vi "BreadBoardLabVIEWtoArduino.vi"() -> ()   [LabVIEW 2024]
uses:
  <vilib>/Instr/_visa.llb/VISA Configure Serial Port (Instr).vi
  <vilib>/Utility/file.llb/Write Delimited Spreadsheet (DBL).vi
  <vilib>/Utility/file.llb/Write Delimited Spreadsheet (string).vi
panel:
  in  "Numeric 2":dbl
  out "Numeric":dbl format="%#_6f"
  in  "file path (dialog if empty)":path
  out "x-y":u32
  out "String":string
  in  "Boolean":bool
  in  "stop":bool
  in  "VISA resource name":refnum<visa-resource-name>
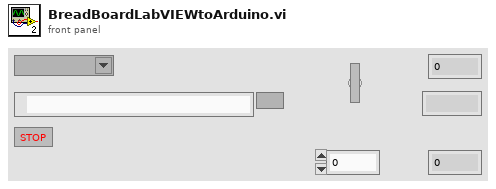
[diagram p1: front panel]
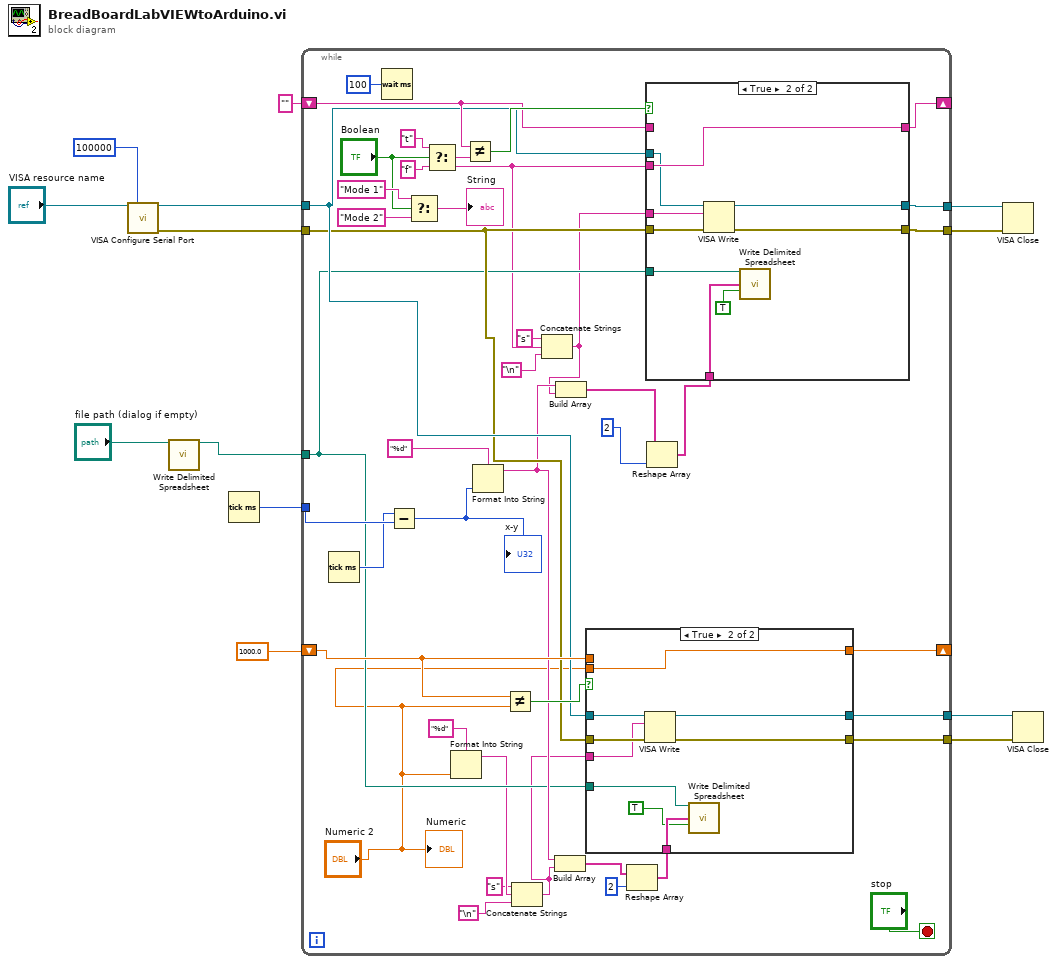
[diagram p0: block diagram]
diagram:
  n1 = call-poly "VISA Configure Serial Port"("VISA resource name"="VISA resource name", "timeout (10sec)"=u32 100000) -> ("VISA resource name out"=w2:refnum<visa-resource-name>, "error out"=w1:errorcluster)  [unwired: 12 in]
  n2 = call-poly <vilib>:"Write Delimited Spreadsheet.vi"("file path (dialog if empty)"="file path (dialog if empty)") -> ("new file path (Not A Path if cancelled)"=w8:path)  [unwired: 13 in, 1 out]
  n3 = Tick Count (ms)() -> (millisecond timer value=w7:u32)
  n4 = while {
    tunnel: w1 -> [w28]
    tunnel: [w48] -> w11
    tunnel: [w47] -> w10
    tunnel: w2 -> [w31]
    shift-right: [w49] -> _
    shift-left: "" -> [w50]
    tunnel: w8 -> [w23]
    tunnel: w7 -> [w40]
    shift-right: [w35] -> _
    shift-left: 1000.0 -> [w34]
    tunnel: [w30] -> w4
    tunnel: [w29] -> w3
    stop <- "stop" stop-if-true
    n5 = Tick Count (ms)() -> (millisecond timer value=w39:u32)
    n6 = Wait (ms)(milliseconds to wait=u32 100) -> ()  [unwired: 1 out]
    n7 = Subtract(x=w39, y=w40) -> (x-y=w41:u32)
    "x-y" <- w41
    n8 = Select(t="Mode 1", s="Boolean", f="Mode 2") -> (s? t:f=→"String":string)
    n9 = Select(t="t", s="Boolean", f="f") -> (s? t:f=w20:string)
    n10 = Format Into String(format string="%d", "Numeric 2") -> (resulting string=w18:string)  [unwired: 2 in, 1 out]
    n11 = Not Equal?(x=w50, y=w20) -> (x != y?=w53:bool)
    n12 = Format Into String(format string="%d", w41) -> (resulting string=w26:string)  [unwired: 2 in, 1 out]
    n13 = Not Equal?(x=w34, y="Numeric 2") -> (x != y?=w33:bool)
    n14 = Concatenate Strings("s" ("string"), w18, "\n") -> (w17:string)
    n15 = Concatenate Strings("s" ("string"), w20, "\n") -> (w21:string)
    n16 = Build Array(w26, w17) -> (w25:string[])
    n17 = Build Array(w26, w21) -> (w38:string[])
    n18 = Reshape Array(w25, 2 ("dimension size")) -> (w24:string[])
    n19 = case shown="True" w33 {
      tunnel: [w58 w67] -> w35
      tunnel: w34 -> [w58 _]
      tunnel: w17 -> [_ w61]
      tunnel: "Numeric 2" -> [_ w67]
      tunnel: w31 -> [w57 w66]
      tunnel: [w57 w60] -> w30
      tunnel: [w56 w59] -> w29
      tunnel: w28 -> [w56 w65]
      tunnel: w24 -> [_ w64]
      tunnel: w23 -> [_ w63]
      frame False {
      }
      frame True {
        n20 = VISA Write(VISA resource name=w66, write buffer=w61, error in (no error)=w65) -> (VISA resource name out=w60:refnum<visa-resource-name>, error out=w59:errorcluster)  [unwired: 1 out]
        n21 = call-poly <vilib>:"Write Delimited Spreadsheet.vi"("file path (dialog if empty)"=w63, "1D data"=w64, "append to file? (new file:F)"=TRUE) -> ()  [unwired: 11 in, 2 out]
      }
    }
    n22 = Reshape Array(w38, 2 ("dimension size")) -> (w36:string[])
    n23 = case shown="True" w53 {
      tunnel: [w70 w79] -> w49
      tunnel: w20 -> [_ w79]
      tunnel: w50 -> [w70 _]
      tunnel: w28 -> [w68 w78]
      tunnel: w31 -> [w69 w77]
      tunnel: [w68 w72] -> w48
      tunnel: [w69 w73] -> w47
      tunnel: w23 -> [_ w76]
      tunnel: w36 -> [_ w74]
      tunnel: w21 -> [_ w71]
      frame False {
      }
      frame True {
        n24 = VISA Write(VISA resource name=w77, write buffer=w71, error in (no error)=w78) -> (VISA resource name out=w73:refnum<visa-resource-name>, error out=w72:errorcluster)  [unwired: 1 out]
        n25 = call-poly <vilib>:"Write Delimited Spreadsheet.vi"("file path (dialog if empty)"=w76, "1D data"=w74, "append to file? (new file:F)"=TRUE) -> ()  [unwired: 11 in, 2 out]
      }
    }
    "Numeric" <- "Numeric 2"
  }
  n26 = VISA Close(VISA resource name=w10, error in (no error)=w11) -> ()  [unwired: 1 out]
  n27 = VISA Close(VISA resource name=w4, error in (no error)=w3) -> ()  [unwired: 1 out]
